vi "UpdateMTsumRTToRT1.vi"() -> ()   [LabVIEW 2012]
uses:
  <vilib>/addons/database/Connection.llb/DB Tools Open Connec (Path).vi
  <vilib>/addons/database/Connection.llb/Conn Execute.vi
  <vilib>/addons/database/Recordset.llb/Rec Destroy - Connection.vi
  <vilib>/addons/database/NI_Database_API.lvlib
panel:
  out "error out":errorcluster
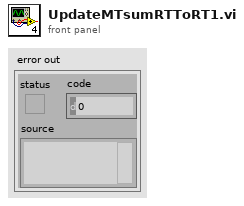
[diagram p1: front panel]
types:
  T1 = typedef "NI_Database_API.lvlib/Conn ObjectReference.ctl" = refnum<k1>
  T2 = typedef "NI_Database_API.lvlib/Rec ObjectReference.ctl" = refnum<k1>
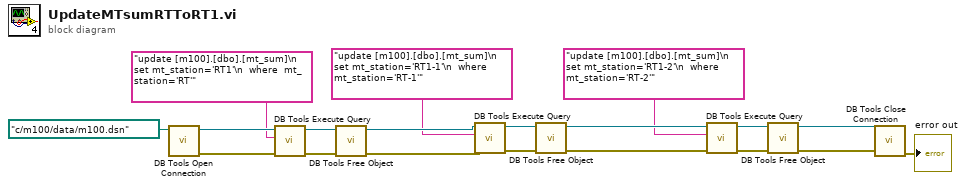
[diagram p0: block diagram]
diagram:
  n1 = call-poly <vilib>:"DB Tools Open Connection.vi"("connection information"=path "c:/m100/data/m100.dsn") -> ("error out"=w18:errorcluster, "connection reference"=w19:T1)  [unwired: 7 in]
  n2 = call-poly <vilib>:"DB Tools Execute Query.vi"("error in (no error)"=w18, "SQL query"="update [m100].[dbo].[mt_sum]\n  set mt_station='RT1'\n  where  mt_station='RT'", "connection reference"=w19) -> ("error out"=w16:errorcluster, "recordset reference"=w17:T2)  [unwired: 5 in]
  n3 = call-poly <vilib>:"DB Tools Free Object.vi"("error in (no error)"=w16, "recordset reference"=w17) -> ("error out"=w10:errorcluster, "connection reference"=w11:T1)  [unwired: 8 in]
  n4 = call-poly <vilib>:"DB Tools Execute Query.vi"("error in (no error)"=w10, "SQL query"="update [m100].[dbo].[mt_sum]\n  set mt_station='RT1-1'\n  where  mt_station='RT-1'", "connection reference"=w11) -> ("error out"=w12:errorcluster, "recordset reference"=w13:T2)  [unwired: 5 in]
  n5 = call-poly <vilib>:"DB Tools Free Object.vi"("error in (no error)"=w12, "recordset reference"=w13) -> ("error out"=w4:errorcluster, "connection reference"=w5:T1)  [unwired: 8 in]
  n6 = call-poly <vilib>:"DB Tools Execute Query.vi"("error in (no error)"=w4, "SQL query"="update [m100].[dbo].[mt_sum]\n  set mt_station='RT1-2'\n  where  mt_station='RT-2'", "connection reference"=w5) -> ("error out"=w6:errorcluster, "recordset reference"=w7:T2)  [unwired: 5 in]
  n7 = call-poly <vilib>:"DB Tools Free Object.vi"("error in (no error)"=w6, "recordset reference"=w7) -> ("error out"=w2:errorcluster, "connection reference"=w3:T1)  [unwired: 8 in]
  n8 = call <vilib>:"DB Tools Close Connection.vi"("error in (no error)"=w2, "connection reference"=w3) -> ("error out"=→"error out":errorcluster)  [unwired: 5 in]
